vi "PatternMatch.vi"(8 "error in":errorcluster, 9 "ROI":T1, 10 "Template":T2, 11 "Image":T2) -> (0 "error out":errorcluster, 1 "Score":sgl, 2 "Attempt":i32, 3 "Position":cluster{"x":sgl, "y":sgl}, 5 "Image 2":T2(plugin-control))   [LabVIEW 2025]
uses:
  <vilib>/vision/Image Controls.llb/IMAQ Image.ctl
  <vilib>/vision/NI_Vision_Development_Module.lvlib
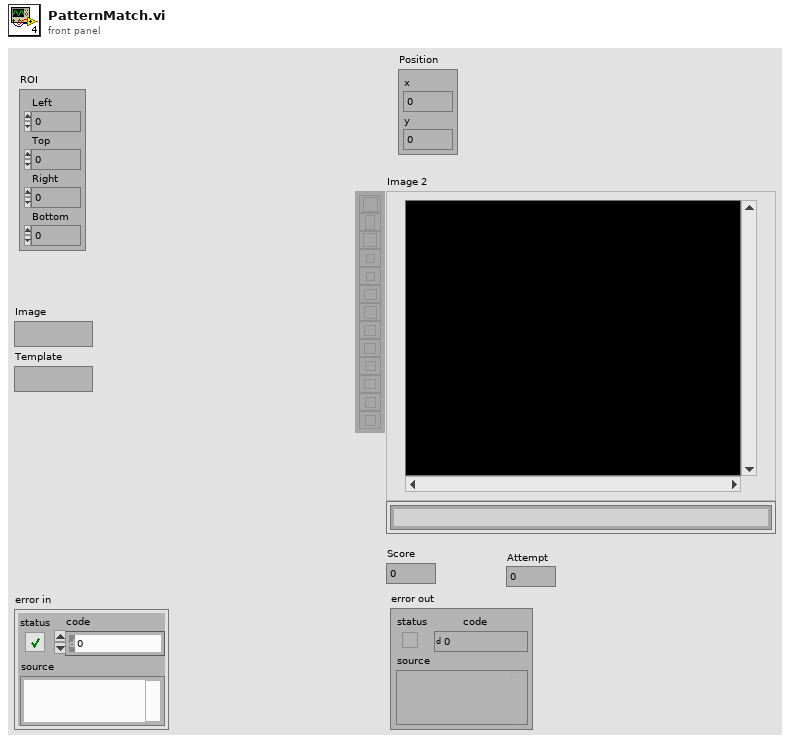
[diagram p1: front panel]
types:
  T1 = cluster{"Left":i32, "Top":i32, "Right":i32, "Bottom":i32}
  T2 = typedef "IMAQ Image.ctl" = refnum<image>
  T3 = typedef "Image Type" = u32
  T4 = cluster{"Show Search Area":bool, "Show Result":bool}
  T5 = cluster{"Position":cluster{"x":sgl, "y":sgl}, "Angle":sgl, "Scale":sgl, "Score":sgl, "Bounding Box":cluster{"x":sgl, "y":sgl}[]}[]
  T6 = cluster{"Position":cluster{"x":sgl, "y":sgl}, "Angle":sgl, "Scale":sgl, "Score":sgl, "Bounding Box":cluster{"x":sgl, "y":sgl}[]}
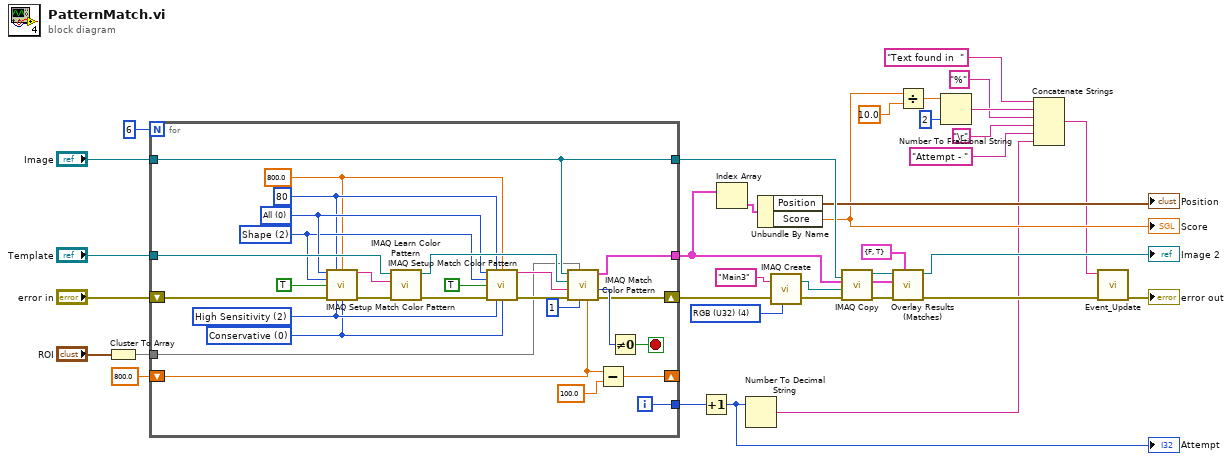
[diagram p0: block diagram]
diagram:
  w29 = T3 4 items=["Grayscale (U8)", "Grayscale (I16)", "Grayscale (SGL)", "Complex (CSG)", "RGB (U32)", "HSL (U32)", "RGB (U64)", "Grayscale (U16)"] ("Image Type")
  n1 = Cluster To Array(cluster="ROI") -> (array=w23:i32[])
  n2 = for {
    N: 6 -> [_]
    tunnel: [w57] -> w25
    tunnel: "Template" -> [w53]
    shift-right: [w55] -> w28
    shift-left: "error in" -> [w54]
    shift-right: [w60] -> _
    shift-left: sgl 800.0 ("Minimum Match Score") -> [w62]
    tunnel: [w58] -> w32
    tunnel: "Image" -> [w37]
    tunnel: [w37] -> w24
    tunnel: w23 -> [w36]
    i -> [w58]
    stop <- w59 stop-if-true
    w38 = u32 0 items=["Conservative", "Balance", "Aggressive", "Very Aggressive"] ("Search Strategy")
    w40 = u32 2 items=["Low Sensitivity", "Medium Sensitivity", "High Sensitivity"] ("Color Sensitivity")
    w41 = 80 ("Minimum Contrast")
    w39 = sgl 800.0 ("Color Score Weight")
    w45 = u32 2 items=["Color and Shape", "Color", "Shape "] ("Feature Mode")
    w46 = u32 0 items=["All", "Shift Information", "Rotation Information"] ("Learn Mode")
    n3 = call "IMAQ Setup Match Color Pattern"("Match Mode"=w46, "Minimum Contrast"=w41, "Color Score Weight"=w39, "Match Feature Mode"=w45, "Subpixel Accuracy"=TRUE, "error in (no error)"=w54, "Color Sensitivity"=w40, "Search Strategy"=w38) -> ("Match Color Pattern Setup Data"=w43:string, "error out"=w47:errorcluster)  [unwired: 6 in]
    n4 = call "IMAQ Learn Color Pattern"("error in (no error)"=w47, "Learn Color Pattern Setup Data"=w43, "Image"=w53) -> ("error out"=w49:errorcluster, "Template Image Out"=w51:T2)  [unwired: 7 in]
    n5 = call "IMAQ Setup Match Color Pattern"("Match Mode"=w46, "Minimum Contrast"=w41, "Color Score Weight"=w39, "Match Feature Mode"=w45, "Subpixel Accuracy"=TRUE, "error in (no error)"=w49, "Color Sensitivity"=w40, "Search Strategy"=w38) -> ("Match Color Pattern Setup Data"=w42:string, "error out"=w48:errorcluster)  [unwired: 6 in]
    n6 = call "IMAQ Match Color Pattern"("Minimum Match Score"=w62, "Number of Matches Requested"=1, "Optional Rectangle"=w36, "error in (no error)"=w48, "Match Color Pattern Setup Data"=w42, "Template Image"=w51, "Image"=w37) -> ("error out"=w55:errorcluster, "Number of Matches"=w56:i32, "Matches"=w57:T5)  [unwired: 2 in]
    n7 = Subtract(x=w62, y=sgl 100.0) -> (x-y=w60:sgl)
    n8 = Not Equal To 0?(x=w56) -> (x != 0?=w59:bool)
  }
  n9 = Increment(x=w32) -> (x+1=w4:i32)
  "Attempt" <- w4
  n10 = Index Array(array=w25) -> (element=w35:T6)  [unwired: 1 in]
  n11 = Number To Decimal String(number=w4) -> (decimal integer string=w2:string)  [unwired: 1 in]
  n12 = Unbundle By Name(w35) -> ("Position"=→"Position":cluster{"x":sgl, "y":sgl}, "Score"=w12:sgl)
  "Score" <- w12
  n13 = call "IMAQ Create"("Image Name"="Main3", "Image Type"=w29, "error in (no error)"=w28) -> ("New Image"=w27:T2, "error out"=w21:errorcluster)  [unwired: 2 in]
  n14 = call "IMAQ Copy"("error in (no error)"=w21, "Image Dst"=w27, "Image Src"=w24) -> ("error out"=w22:errorcluster, "Image Dst Out"=w26:T2)  [unwired: 3 in]
  n15 = call <vilib>:"Overlay Results (Matches).vi"("Setup"=T4 {"Show Search Area"=FALSE, "Show Result"=TRUE}, "error in"=w22, "Matches"=w25, "Image In"=w26) -> ("error out"=w14:errorcluster, "Image Out"=→"Image 2":T2)  [unwired: 2 in, 4 out]
  n16 = Divide(x=w12, y=sgl 10.0) -> (x/y=w9:sgl)
  n17 = Number To Fractional String(number=w9, precision (6)=i16 2) -> (F-format string=w7:string)  [unwired: 2 in]
  n18 = Concatenate Strings("Text found in  " ("Image Name"), w7, "%", "\r", "Attempt - ", w2) -> (w5:string)
  n19 = call "Event_Update.vi"("Error In"=w14, "Event"=w5) -> ("Error Out"=→"error out":errorcluster)  [unwired: 9 in]
